vi "Remove From Tree If Filtered.vi"(8 "error in (no error)":errorcluster, 10 "Not Found":string[](array[string]), 11 "TreeControl in":refnum<vi>) -> (0 "error out":errorcluster)   [LabVIEW 2013, in "FindName Task_Manager.lvlib"]
uses:
  FindName Task_Manager.lvlib
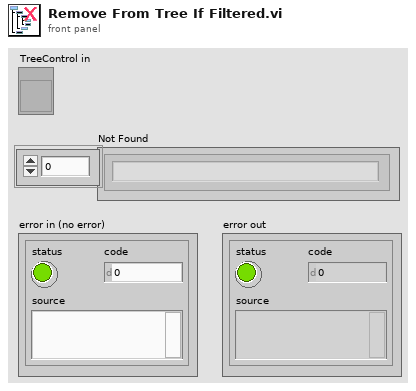
[diagram p1: front panel]
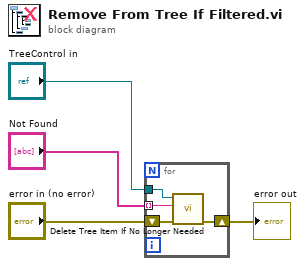
[diagram p0: block diagram]
diagram:
  n1 = for {
    tunnel: "Not Found" -> [w8] mode=indexing
    shift-right: [w7] -> w2
    shift-left: "error in (no error)" -> [w6]
    tunnel: "TreeControl in" -> [w5]
    n2 = call "Delete Tree Item If No Longer Needed.vi"("error in"=w6, "Item Tag"=w8, "Tree Ref"=w5) -> ("error out"=w7:errorcluster)  [unwired: 8 in]
  }
  "error out" <- w2
